vi "Webcam_trial.vi"() -> ()   [LabVIEW 2017]
uses:
  <vilib>/imath/engines/lvmath2/RunTimeEngine/Managers/WorkSpace/UID Generator.vi
  <vilib>/imath/engines/lvmath2/RunTimeEngine/RunTimeType/NIMS_RunTimeType_From StrictType (excl LVString).vi
  <instcachedir>/0/NIMS_RunTimeType_From StrictType (excl LVString)_1019F277F0A747EDBCA0F6C52CA54500.lvgen/NIMS_RunTimeType_From StrictType (excl LVString)_1019F277F0A747EDBCA0F6C52CA54500_000.vi
  <vilib>/imath/engines/lvmath2/RunTimeEngine/LocalVariableDefStatement/MC_LocalVariableDefStatement_Display.vi
  <vilib>/imath/engines/lvmath2/RunTimeEngine/RangeToken/NIMS_Range.vi
  <instcachedir>/0/NIMS_Range_69CB9AAD882742A19CF7E739BE79952C.lvgen/NIMS_Range_69CB9AAD882742A19CF7E739BE79952C_000.vi
  <vilib>/imathl/engines/lvmath/Functions/Error Handling/Create Error.vi
  <vilib>/imath/engines/lvmath2/RunTimeEngine/Managers/SymbolTable/Clear UID.vi
  <vilib>/imath/engines/lvmath2/RunTimeEngine/NodeEndStatement/NIMS_NodeEndStatement_Output.vi
  <instcachedir>/0/NIMS_NodeEndStatement_Output_53EC0D466D134D7ABD903AC30B43404B.lvgen/NIMS_NodeEndStatement_Output_53EC0D466D134D7ABD903AC30B43404B_005.vi
  <vilib>/imath/engines/lvmath2/RunTimeEngine/ErrorHandling/NIMS_Finalize Error.vi
  <vilib>/imath/engines/lvmath2/RunTimeEngine/Managers/SymbolTable/NIMS_WorkSpace.lvlib
panel:
  out "Array 2":u32[][](array[colorbox])
  in  "Array":u32[][](array[colorbox])=[[0, 0, 0, 0, 0, 0, 0, 0, 0, 0], [0, 0, 0, 0, 0, 0, 0, 0, 0, 0], [0, 0, 0, 0, 0, 0, 0, 0, 0, 0], [0, 0, 0, 0, 0, 0, 0, 0, 0, 0], [0, 0, 0, 0, 0, 0, 0, 0, 0, 0], [0, 0, 0, 0, 0, 0, 0, 0, 0, 0], [0, 0, 0, 0, 0, 0, 0, 0, 0, 65793]]
  out "appended array 2":dbl[](array[numeric])
  out "appended array":dbl[][](array[numeric])
  out "cluster":T1
  out "array w/ subset deleted":dbl[](array[numeric])
  out "Waveform Graph":cluster{dbl, dbl, "x":dbl[]}(graph)
  out "Waveform Chart":dbl[](graph)
  out "x":dbl[](array[numeric])
  out "t":dbl[](array[numeric])
  in  "Digitizing Parameters":T2={"Numbers of Samples"=100, "Sampling Frequency"=1000.0}
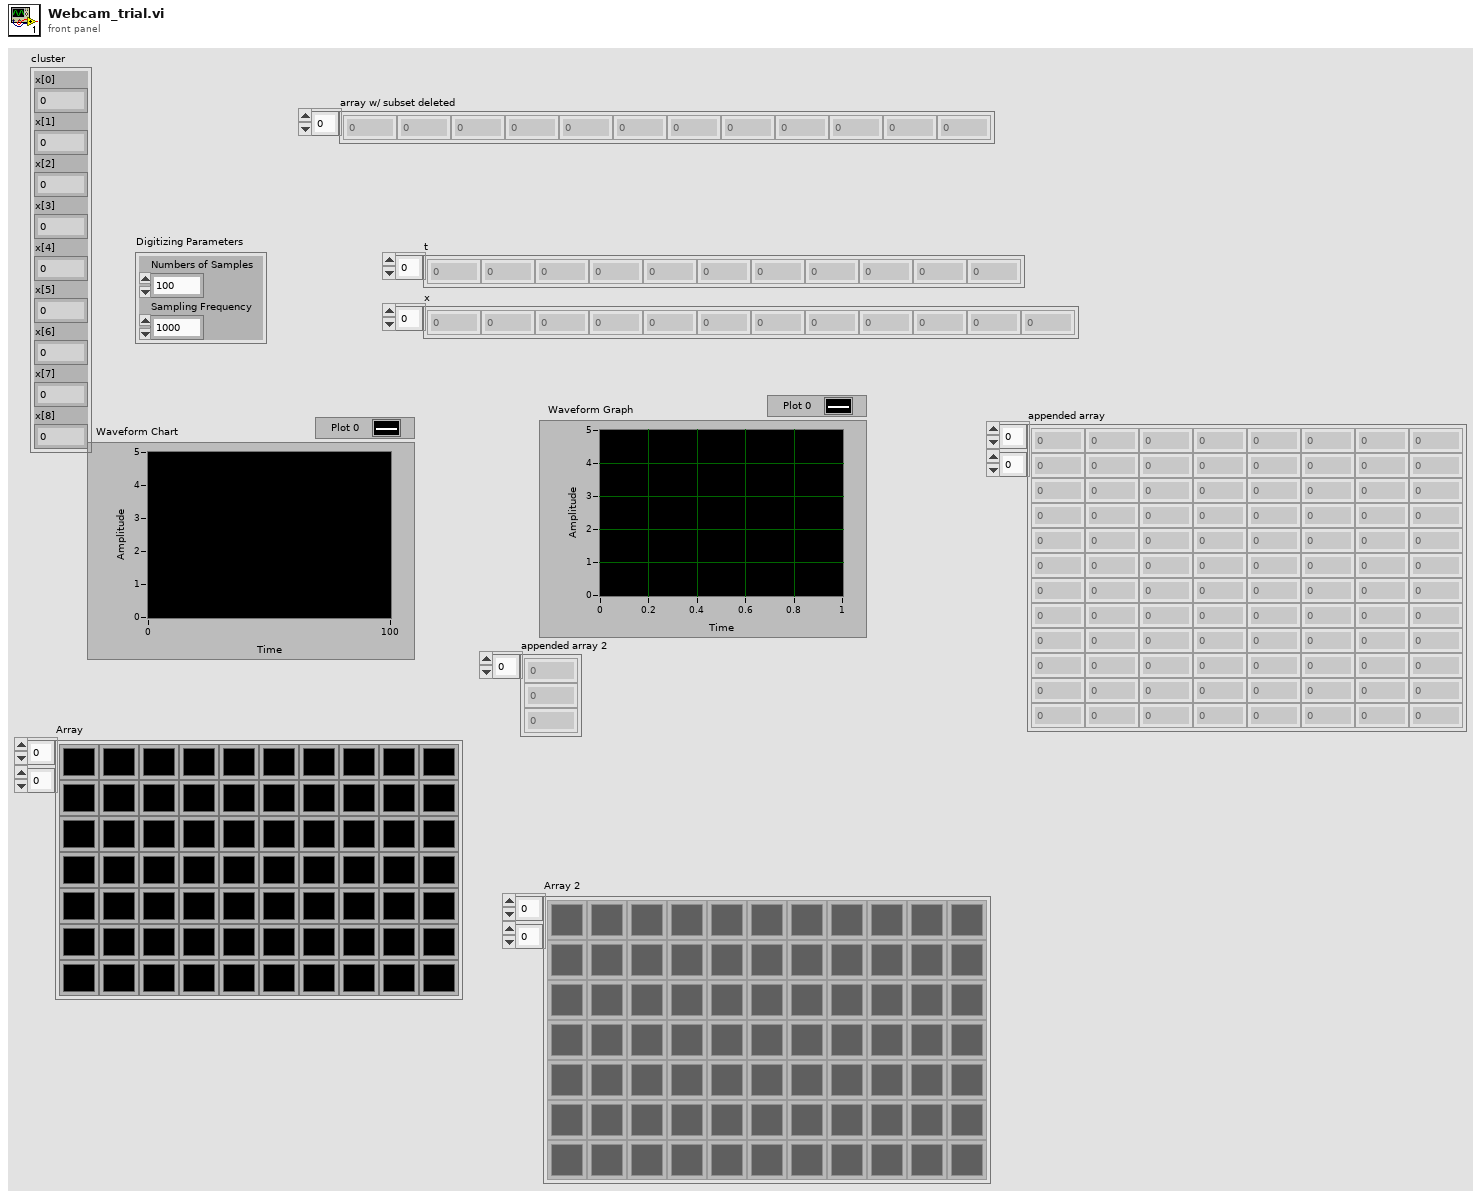
[diagram p1: front panel]
types:
  T1 = cluster{"x[0]":dbl, "x[1]":dbl, "x[2]":dbl, "x[3]":dbl, "x[4]":dbl, "x[5]":dbl, "x[6]":dbl, "x[7]":dbl, "x[8]":dbl}
  T2 = cluster{"Numbers of Samples":i32, "Sampling Frequency":dbl}
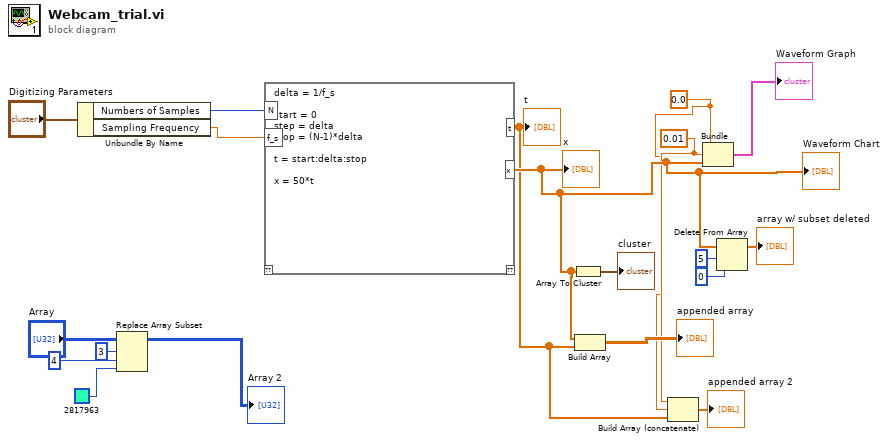
[diagram p0: block diagram]
diagram:
  w9 = 0.01
  w8 = 0.0
  n1 = Unbundle By Name("Digitizing Parameters") -> ("Numbers of Samples"=w17:i32, "Sampling Frequency"=w18:dbl)
  n2 = Replace Array Subset(array="Array", new element=u32 2817963, index (row)=3, index (col)=4 ("disabled index (col)")) -> (→"Array 2":u32[][])
  n3 = mathscript code="delta = 1/f_s\n\nstart = 0\nstep = delta\nstop = (N-1)*delta\n\nt = start:delta:stop\n\nx = 50*t"("N"=w17, "f_s"=w18) -> ("t"=w7:dbl[], "x"=w11:dbl[])  [unwired: 1 in, 1 out]
  "t" <- w7
  "x" <- w11
  "Waveform Chart" <- w11
  n4 = Array To Cluster(array=w11) -> (cluster=→"cluster":T1)
  n5 = Build Array(w11, w7) -> (→"appended array":dbl[][])
  n6 = Build Array (concatenate)(w9, w8, w7) -> (→"appended array 2":dbl[])
  n7 = Bundle(w8, w9, "x"=w11) -> (→"Waveform Graph":cluster{dbl, dbl, "x":dbl[]})  [unwired: 1 in]
  n8 = Delete From Array(array=w11, length=5, index=0) -> (array with subset deleted=→"array w/ subset deleted":dbl[])  [unwired: 1 out]
